vi "Edge Detection-2.vi"(8 "error in":errorcluster, 11 "Image":T1) -> (0 "error out":errorcluster, 1 "Particle Variables":i32[](array[ring]) items=["Center of Mass X", "Center of Mass Y", "First Pixel X", "First Pixel Y", "Bounding Rect Left", "Bounding Rect Top", "Bounding Rect Right", "Bounding Rect Bottom", "Max Feret Diameter Start X", "Max Feret Diameter Start Y", "Max Feret Diameter End X", "Max Feret Diameter End Y", "Max Horiz. Segment Length Left", "Max Horiz. Segment Length Right", "Max Horiz. Segment Length Row", "-", "Bounding Rect Width", "Bounding Rect Height", "Bounding Rect Diagonal", "Perimeter", "Convex Hull Perimeter", "Holes' Perimeter", "Max Feret Diameter", "Equivalent Ellipse Major Axis", "Equivalent Ellipse Minor Axis", "Equivalent Ellipse Minor Axis (Feret)", "Equivalent Rect Long Side", "Equivalent Rect Short Side", "Equivalent Rect Diagonal", "Equivalent Rect Short Side (Feret)", "Average Horiz. Segment Length", "Average Vert. Segment Length", "Hydraulic Radius", "Waddel Disk Diameter", "-", "Area", "Holes' Area", "Particle & Holes' Area", "Convex Hull Area", "Image Area", "-", "Number of Holes", "Number of Horiz. Segments", "Number of Vert. Segments", "-", "Orientation", "Max Feret Diameter Orientation", "-", "% Area/Image Area", "% Area/(Particle & Holes' Area)", "Ratio of Equivalent Ellipse Axes", "Ratio of Equivalent Rect Sides", "-", "Elongation Factor", "Compactness Factor", "Heywood Circularity Factor", "Type Factor", "-", "Sum X", "Sum Y", "Sum XX", "Sum XY", "Sum YY", "Sum XXX", "Sum XXY", "Sum XYY", "Sum YYY", "-", "Moment of Inertia XX", "Moment of Inertia XY", "Moment of Inertia YY", "Moment of Inertia XXX", "Moment of Inertia XXY", "Moment of Inertia XYY", "Moment of Inertia YYY", "Norm. Moment of Inertia XX", "Norm. Moment of Inertia XY", "Norm. Moment of Inertia YY", "Norm. Moment of Inertia XXX", "Norm. Moment of Inertia XXY", "Norm. Moment of Inertia XYY", "Norm. Moment of Inertia YYY", "Hu Moment 1", "Hu Moment 2", "Hu Moment 3", "Hu Moment 4", "Hu Moment 5", "Hu Moment 6", "Hu Moment 7"], 2 "Particle Measurements (Pixels)":dbl[][](array[numeric]) format="%.2f", 3 "Image Out":T1(plugin-control), 5 "Number of Particles":i32)   [LabVIEW 2014]
uses:
  <vilib>/vision/Image Controls.llb/IMAQ Image.ctl
  <vilib>/vision/Measure.llb/Edge Options.ctl
  <vilib>/vision/Measure.llb/Edge Polarity.ctl
  FileIO/TypeDef - File Actions.ctl
  <vilib>/vision/NI_Vision_Development_Module.lvlib
panel:
  in  "Display delay (s)":dbl min=0.0 max=5.0 step=0.5
  out "Task":string
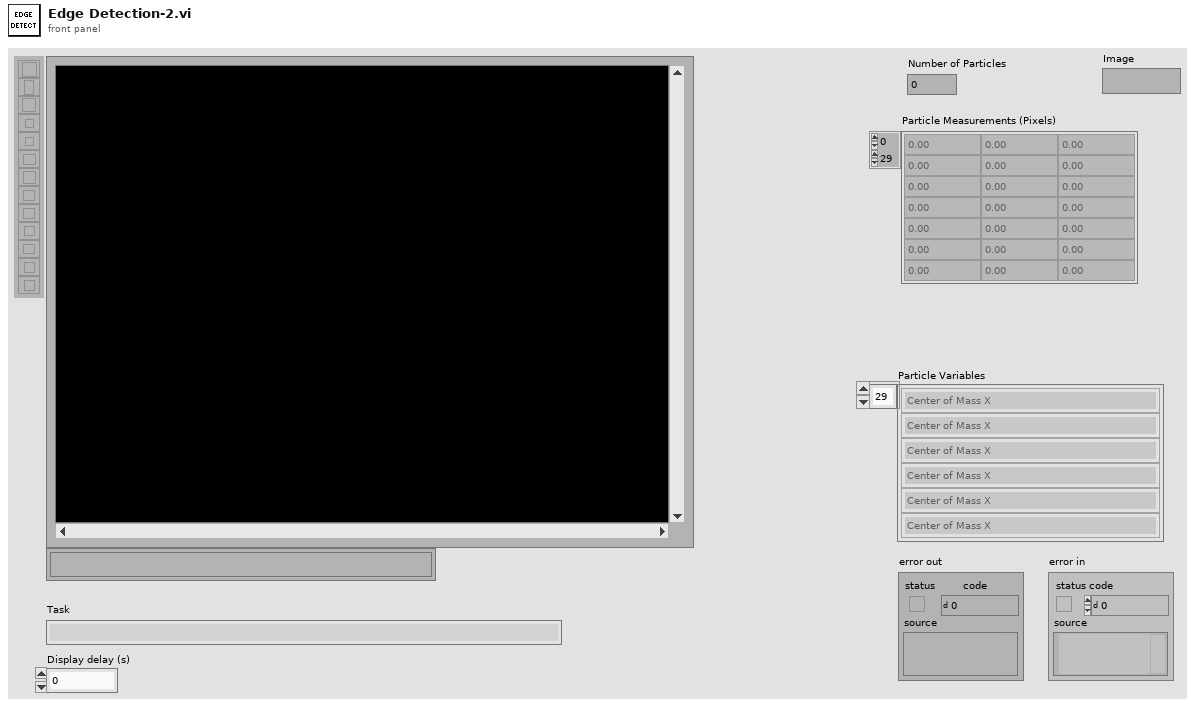
[diagram p1: front panel]
types:
  T1 = typedef "IMAQ Image.ctl" = refnum<image>
  T2 = enum32{"AutoM", "Close", "Dilate", "Erode", "Gradient", "Gradient out", "Gradient in", "Hit miss", "Open", "PClose", "POpen", "Thick", "Thin"}
  T3 = typedef "TypeDef - File Actions.ctl" = enum16{"Read", "Write", "Get Current"}
  T4 = cluster{"Measurement Parameter":i32, "Range Lower Value":dbl, "Range Upper Value":dbl, "Range":bool, "Measurement Type":bool}
  T5 = typedef "Image Type" = u32
  T6 = typedef "Edge Options.ctl" = cluster{"Edge Polarity":T7, "Kernel Size":u32, "Width":u32, "Minimum Edge Strength":sgl, "Interpolation Type":enum32{"Zero Order", "Bilinear", "Quadratic", "Cubic", "Bilinear Fixed"}, "Data Processing Method":enum32{"Average", "Median"}}
  T7 = typedef "Edge Polarity.ctl" = u32
  T8 = cluster{"Search  Direction":u32, "Edge Options":T6, "Show Search Area":bool, "Show Search Lines":bool, "Show Edges Found":bool, "Show Result":bool, "Search Area Color":u32, "Search Lines Color":u32, "Edge Locations Color":u32, "Result Color":u32, "Overlay Group Name":string}
  T9 = cluster{"Process":enum16{"Get First Edge", "Get First + Last Edge", "Get All Edges", "Get Best Edge"}, "Step Size":i32, "Max Pixel Radius":i32}
  T10 = cluster{"Global Rectangle":i32[], "Contours":cluster{"ID":enum32{"External", "Internal"}, "Type":u32, "Coordinates":i32[]}[]}
  T11 = enum32{"Differentiation", "Gradient", "Prewitt", "Roberts", "Sigma", "Sobel"}
  T12 = enum32{"Invalid", "Standard", "Closed", "Hidden", "Minimized", "Maximized"}
  T13 = typedef "TypeDef - System Configuration.ctl" = cluster{"Results FilePath":path, "Analysis Parameters":cluster{"Area":cluster{"Lower Value":dbl, "Upper Value":dbl}, "Circle Filter Radius":cluster{"Lower Value":sgl, "Upper Value":sgl}, "Edge Detection Threshold":u16}, "ROI Parameters":cluster{"ROI size (in Radius)":cluster{"Width":dbl, "Height":dbl}}}
  T14 = cluster{"Center (Pixels)":cluster{"X":sgl, "Y":sgl}, "Radius (Pixels)":dbl, "Center (Real-World)":cluster{"X":sgl, "Y":sgl}, "Radius (Real-World)":dbl, "Roundness (Real-World)":dbl, "Average Strength":dbl, "Average SNR (dB)":dbl}
  T15 = cluster{"Measurement Parameter":i32, "Range Lower Value":dbl, "Range Upper Value":dbl, "Range":bool, "Measurement Type":bool}[]
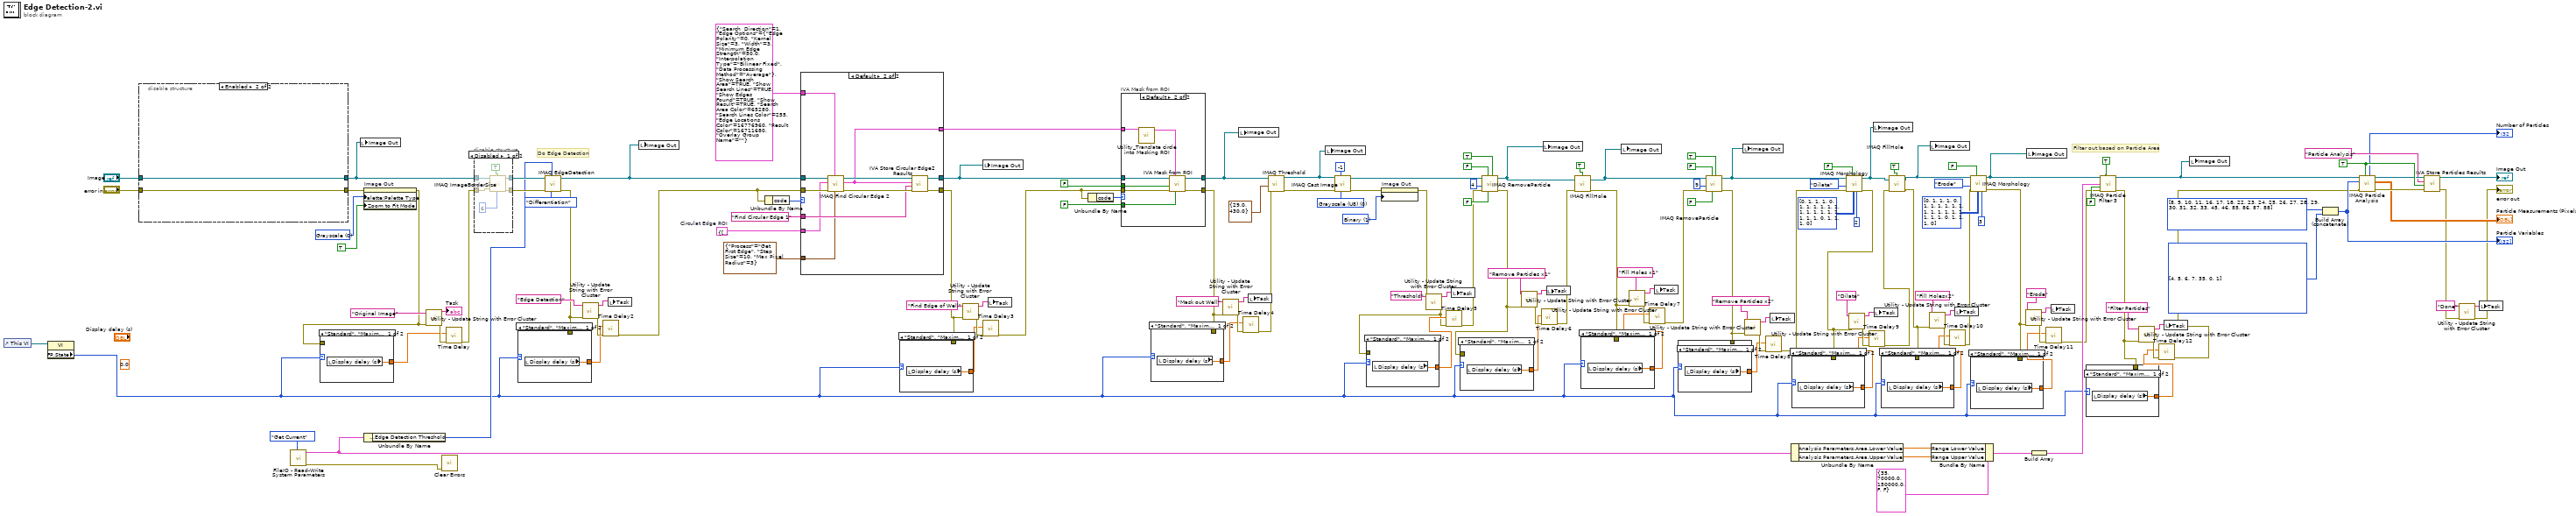
[diagram p0: block diagram]
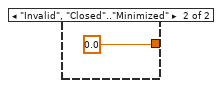
[diagram p2: hidden frame]
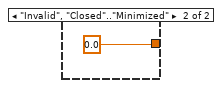
[diagram p3: hidden frame]
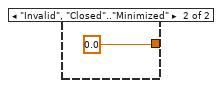
[diagram p4: hidden frame]
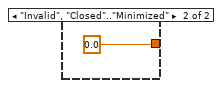
[diagram p5: hidden frame]
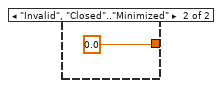
[diagram p6: hidden frame]
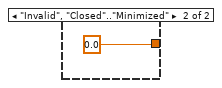
[diagram p7: hidden frame]
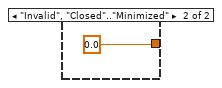
[diagram p8: hidden frame]
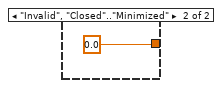
[diagram p9: hidden frame]
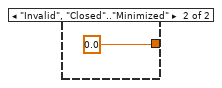
[diagram p10: hidden frame]
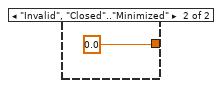
[diagram p11: hidden frame]
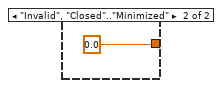
[diagram p12: hidden frame]
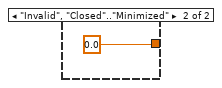
[diagram p13: hidden frame]
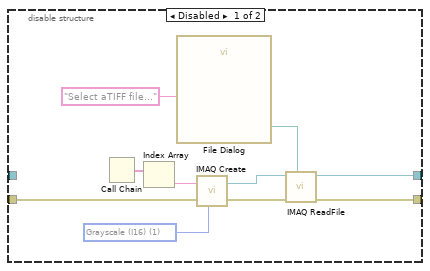
[diagram p16: hidden frame]
diagram:
  (unwired) 0.0 ("f")
  w108 = i32[] [4, 5, 6, 7, 35, 0, 1] items=["Center of Mass X", "Center of Mass Y", "First Pixel X", "First Pixel Y", "Bounding Rect Left", "Bounding Rect Top", "Bounding Rect Right", "Bounding Rect Bottom", "Max Feret Diameter Start X", "Max Feret Diameter Start Y", "Max Feret Diameter End X", "Max Feret Diameter End Y", "Max Horiz. Segment Length Left", "Max Horiz. Segment Length Right", "Max Horiz. Segment Length Row", "-", "Bounding Rect Width", "Bounding Rect Height", "Bounding Rect Diagonal", "Perimeter", "Convex Hull Perimeter", "Holes' Perimeter", "Max Feret Diameter", "Equivalent Ellipse Major Axis", "Equivalent Ellipse Minor Axis", "Equivalent Ellipse Minor Axis (Feret)", "Equivalent Rect Long Side", "Equivalent Rect Short Side", "Equivalent Rect Diagonal", "Equivalent Rect Short Side (Feret)", "Average Horiz. Segment Length", "Average Vert. Segment Length", "Hydraulic Radius", "Waddel Disk Diameter", "-", "Area", "Holes' Area", "Particle & Holes' Area", "Convex Hull Area", "Image Area", "-", "Number of Holes", "Number of Horiz. Segments", "Number of Vert. Segments", "-", "Orientation", "Max Feret Diameter Orientation", "-", "% Area/Image Area", "% Area/(Particle & Holes' Area)", "Ratio of Equivalent Ellipse Axes", "Ratio of Equivalent Rect Sides", "-", "Elongation Factor", "Compactness Factor", "Heywood Circularity Factor", "Type Factor", "-", "Sum X", "Sum Y", "Sum XX", "Sum XY", "Sum YY", "Sum XXX", "Sum XXY", "Sum XYY", "Sum YYY", "-", "Moment of Inertia XX", "Moment of Inertia XY", "Moment of Inertia YY", "Moment of Inertia XXX", "Moment of Inertia XXY", "Moment of Inertia XYY", "Moment of Inertia YYY", "Norm. Moment of Inertia XX", "Norm. Moment of Inertia XY", "Norm. Moment of Inertia YY", "Norm. Moment of Inertia XXX", "Norm. Moment of Inertia XXY", "Norm. Moment of Inertia XYY", "Norm. Moment of Inertia YYY", "Hu Moment 1", "Hu Moment 2", "Hu Moment 3", "Hu Moment 4", "Hu Moment 5", "Hu Moment 6", "Hu Moment 7"] ("Pixel Measurements")
  w111 = u32 0 items=["Grayscale", "Binary", "Gradient", "Rainbow", "Temperature", "User Defined"] ("Palette")
  w121 = u32 1 items=["Grayscale", "Binary", "Gradient", "Rainbow", "Temperature", "User Defined"] ("Palette")
  w109 = i32[] [8, 9, 10, 11, 16, 17, 18, 22, 23, 24, 25, 26, 27, 28, 29, 30, 31, 32, 33, 45, 46, 85, 86, 87, 88] items=["Center of Mass X", "Center of Mass Y", "First Pixel X", "First Pixel Y", "Bounding Rect Left", "Bounding Rect Top", "Bounding Rect Right", "Bounding Rect Bottom", "Max Feret Diameter Start X", "Max Feret Diameter Start Y", "Max Feret Diameter End X", "Max Feret Diameter End Y", "Max Horiz. Segment Length Left", "Max Horiz. Segment Length Right", "Max Horiz. Segment Length Row", "-", "Bounding Rect Width", "Bounding Rect Height", "Bounding Rect Diagonal", "Perimeter", "Convex Hull Perimeter", "Holes' Perimeter", "Max Feret Diameter", "Equivalent Ellipse Major Axis", "Equivalent Ellipse Minor Axis", "Equivalent Ellipse Minor Axis (Feret)", "Equivalent Rect Long Side", "Equivalent Rect Short Side", "Equivalent Rect Diagonal", "Equivalent Rect Short Side (Feret)", "Average Horiz. Segment Length", "Average Vert. Segment Length", "Hydraulic Radius", "Waddel Disk Diameter", "-", "Area", "Holes' Area", "Particle & Holes' Area", "Convex Hull Area", "Image Area", "-", "Number of Holes", "Number of Horiz. Segments", "Number of Vert. Segments", "-", "Orientation", "Max Feret Diameter Orientation", "-", "% Area/Image Area", "% Area/(Particle & Holes' Area)", "Ratio of Equivalent Ellipse Axes", "Ratio of Equivalent Rect Sides", "-", "Elongation Factor", "Compactness Factor", "Heywood Circularity Factor", "Type Factor", "-", "Sum X", "Sum Y", "Sum XX", "Sum XY", "Sum YY", "Sum XXX", "Sum XXY", "Sum XYY", "Sum YYY", "-", "Moment of Inertia XX", "Moment of Inertia XY", "Moment of Inertia YY", "Moment of Inertia XXX", "Moment of Inertia XXY", "Moment of Inertia XYY", "Moment of Inertia YYY", "Norm. Moment of Inertia XX", "Norm. Moment of Inertia XY", "Norm. Moment of Inertia YY", "Norm. Moment of Inertia XXX", "Norm. Moment of Inertia XXY", "Norm. Moment of Inertia XYY", "Norm. Moment of Inertia YYY", "Hu Moment 1", "Hu Moment 2", "Hu Moment 3", "Hu Moment 4", "Hu Moment 5", "Hu Moment 6", "Hu Moment 7"] ("Pixel Measurements")
  w125 = TRUE ("Connectivity 4/8 (8)")
  w141 = T5 0 items=["Grayscale (U8)", "Grayscale (I16)", "Grayscale (SGL)", "Complex (CSG)", "RGB (U32)", "HSL (U32)", "RGB (U64)", "Grayscale (U16)"] ("Image Type")
  w148 = T10 {"Global Rectangle"=[18, -169, 2540, 2352], "Contours"=[{"ID"=enum."External", "Type"=7, "Coordinates"=[1278, 1091, 691, 1260, 0, 359834]}]}  # Circulat Edge ROI
  # "Do Edge Detection"
  # "Filter out based on Particle Area"
  n1 = control-ref of="This VI"() -> (w80:refnum<vi>)
  n2 = property class="VI"(reference=w80) -> ("FP.State"=w3:T12)  [unwired: 1 in, 2 out]
  n3 = disable-structure shown="Enabled" {
    disable-tunnel: [w163 w165] -> w104
    disable-tunnel: "error in" -> [w161 w165]
    disable-tunnel: [w155 w164] -> w120
    disable-tunnel: "Image" -> [_ w164]
    frame Disabled {
      w156 = T5 1 items=["Grayscale (U8)", "Grayscale (I16)", "Grayscale (SGL)", "Complex (CSG)", "RGB (U32)", "HSL (U32)", "RGB (U64)", "Grayscale (U16)"] ("Image Type")
      n4 = Call Chain() -> (call chain=w160:string[])
      n5 = Index Array(array=w160) -> (element=w159:string)  [unwired: 1 in]
      n6 = call "File Dialog"("prompt"="Select aTIFF file...") -> ("selected path"=w157:path)  [unwired: 6 in, 8 out]
      n7 = call "IMAQ Create"("Image Name"=w159, "Image Type"=w156, "error in (no error)"=w161) -> ("New Image"=w162:T1, "error out"=w154:errorcluster)  [unwired: 1 in, 1 out]
      n8 = call "IMAQ ReadFile"("File Path"=w157, "error in (no error)"=w154, "Image"=w162) -> ("error out"=w163:errorcluster, "Image Out"=w155:T1)  [unwired: 2 in, 5 out]
    }
    frame Enabled {
    }
  }
  n9 = call "FileIO - Read-Write System Parameters.vi"("Action"=TypeDef_-_File_Actions."Get Current") -> ("error out"=w96:errorcluster, "System Parameters out"=w18:T13)  [unwired: 9 in]
  n10 = local write "Image Out"(w120) -> ()
  n11 = property on="Image Out" class="ImageControl"(error in=w104, "Palette:Palette Type"=w111, "Zoom to Fit Mode"=TRUE) -> (error out=w27:errorcluster)  [unwired: 1 in, 1 out]
  n12 = case shown="\"Standard\", \"Maximized\"" w3 {
    tunnel: [w166 0.0 ("f")] -> w26
    tunnel: w27 -> [_ _]
    frame "Standard", "Maximized" {
      n13 = local read "Display delay (s)"() -> (w166:dbl)
    }
    frame "Invalid", "Closed".."Minimized" {
    }
  }
  n14 = Unbundle By Name(w18) -> ("Analysis Parameters.Edge Detection Threshold"=w16:u16)
  n15 = call "Utility - Update String with Error Cluster.vi"("error in (no error)"=w27, "String In"="Original Image" ("Task")) -> ("error out"=w76:errorcluster, "String Out"=→"Task":string)  [unwired: 8 in]
  n16 = call <vilib>:"Clear Errors.vi"("error in (no error)"=w96) -> ()  [unwired: 5 in, 2 out]
  n17 = call "Time Delay"("error in (no error)"=w76, "Delay Time (s)"=w26) -> ("error out"=w79:errorcluster)  [unwired: 9 in]
  n18 = disable-structure shown="Disabled" {
    disable-tunnel: [w173 w174] -> w152
    disable-tunnel: [w170 w175] -> w150
    disable-tunnel: w120 -> [w169 w175]
    disable-tunnel: w79 -> [w168 w174]
    frame Disabled {
      n19 = call "IMAQ ImageBorderSize"("Get/Set Status? (Set)"=TRUE, "Image"=w169, "Image border size in"=6 ("Border Size"), "error in (no error)"=w168) -> ("Image Out"=w170:T1, "error out"=w173:errorcluster)  [unwired: 1 out]
    }
    frame Enabled {
    }
  }
  n20 = call "IMAQ EdgeDetection"("Method"=T11."Differentiation", "Threshold Value"=w16, "error in (no error)"=w152, "Image Src"=w150) -> ("error out"=w25:errorcluster, "Image Dst Out"=w119:T1)  [unwired: 2 in, 4 out]
  n21 = case shown="\"Standard\", \"Maximized\"" w3 {
    tunnel: [w176 0.0 ("f")] -> w17
    tunnel: w25 -> [_ _]
    frame "Standard", "Maximized" {
      n22 = local read "Display delay (s)"() -> (w176:dbl)
    }
    frame "Invalid", "Closed".."Minimized" {
    }
  }
  n23 = call "Utility - Update String with Error Cluster.vi"("error in (no error)"=w25, "String In"="Edge Detection") -> ("error out"=w75:errorcluster, "String Out"=w73:string)  [unwired: 8 in]
  n24 = call "Time Delay2"("error in (no error)"=w75, "Delay Time (s)"=w17) -> ("error out"=w74:errorcluster)  [unwired: 9 in]
  n25 = local write "Task"(w73) -> ()
  n26 = local write "Image Out"(w119) -> ()
  n27 = Unbundle By Name(w74) -> ("code"=w147:i32)
  n28 = case shown="Default" w147 {
    tunnel: T8 {"Search  Direction"=1, "Edge Options"={"Edge Polarity"=0, "Kernel Size"=3, "Width"=3, "Minimum Edge Strength"=50.0, "Interpolation Type"=enum."Bilinear Fixed", "Data Processing Method"=enum."Average"}, "Show Search Area"=TRUE, "Show Search Lines"=TRUE, "Show Edges Found"=TRUE, "Show Result"=TRUE, "Search Area Color"=65280, "Search Lines Color"=255, "Edge Locations Color"=16776960, "Result Color"=16711680, "Overlay Group Name"=""} ("Options") -> [_ w179]
    tunnel: w119 -> [w178 w189]
    tunnel: w74 -> [_ w188]
    tunnel: [_ w186] -> w23
    tunnel: [w178 w184] -> w118
    tunnel: "Find Circular Edge 1" ("Step Name") -> [_ w183]
    tunnel: w148 -> [_ w182]
    tunnel: T9 {"Process"=enum."Get First Edge", "Step Size"=10, "Max Pixel Radius"=3} ("Circle Fit Options") -> [_ w181]
    tunnel: [_ w180] -> w90
    frame -1074396199, -1074396198 {
      # "Discard Coordinate System Error"
    }
    frame Default {
      n29 = call "IMAQ Find Circular Edge 2"("Circle Fit Options"=w181, "Options"=w179, "error in (no error)"=w188, "ROI Descriptor"=w182, "Image"=w189) -> ("error out"=w187:errorcluster, "Fitted Circle"=w180:T14, "Image Out"=w185:T1)  [unwired: 1 in, 3 out]
      n30 = call <vilib>:"IVA Store Circular Edge2 Results.vi"("error in (no error)"=w187, "Step Name"=w183, "Fitted Circle"=w180, "Image in"=w185) -> ("error out"=w186:errorcluster, "Image dup"=w184:T1)  [unwired: 2 in, 4 out]
    }
  }
  n31 = case shown="\"Standard\", \"Maximized\"" w3 {
    tunnel: [w190 0.0 ("f")] -> w24
    tunnel: w23 -> [_ _]
    frame "Standard", "Maximized" {
      n32 = local read "Display delay (s)"() -> (w190:dbl)
    }
    frame "Invalid", "Closed".."Minimized" {
    }
  }
  n33 = call "Utility - Update String with Error Cluster.vi"("error in (no error)"=w23, "String In"="Find Edge of Well") -> ("error out"=w70:errorcluster, "String Out"=w71:string)  [unwired: 8 in]
  n34 = local write "Image Out"(w118) -> ()
  n35 = call "Time Delay3"("error in (no error)"=w70, "Delay Time (s)"=w24) -> ("error out"=w69:errorcluster)  [unwired: 9 in]
  n36 = local write "Task"(w71) -> ()
  n37 = Unbundle By Name(w69) -> ("code"=w91:i32)
  n38 = case "IVA Mask from ROI" shown="Default" w91 {
    tunnel: w90 -> [_ w194]
    tunnel: FALSE ("Shrink") -> [_ w200]
    tunnel: w118 -> [w192 w199]
    tunnel: w69 -> [_ w198]
    tunnel: [_ w197] -> w22
    tunnel: [w192 w196] -> w117
    tunnel: FALSE ("Out / In") -> [_ w195]
    frame -1074396199, -1074396198 {
      # "Discard\nCoordinate\nSystem\nError"
    }
    frame Default {
      n39 = call "Utility_Translate circle into Masking ROI.vi"("Fitted Circle"=w194) -> ("ROI Descriptor"=w193:T10)  [unwired: 10 in]
      n40 = call <vilib>:"IVA Mask from ROI.vi"("Shrink"=w200, "ROI Descriptor"=w193, "error in (no error)"=w198, "Out / In"=w195, "Image Src"=w199) -> ("error out"=w197:errorcluster, "Image Out"=w196:T1)  [unwired: 5 out]
    }
  }
  n41 = case shown="\"Standard\", \"Maximized\"" w3 {
    tunnel: [w201 0.0 ("f")] -> w21
    tunnel: w22 -> [_ _]
    frame "Standard", "Maximized" {
      n42 = local read "Display delay (s)"() -> (w201:dbl)
    }
    frame "Invalid", "Closed".."Minimized" {
    }
  }
  n43 = call "Utility - Update String with Error Cluster.vi"("error in (no error)"=w22, "String In"="Mask out Well") -> ("error out"=w66:errorcluster, "String Out"=w65:string)  [unwired: 8 in]
  n44 = local write "Image Out"(w117) -> ()
  n45 = call "Time Delay4"("error in (no error)"=w66, "Delay Time (s)"=w21) -> ("error out"=w64:errorcluster)  [unwired: 9 in]
  n46 = local write "Task"(w65) -> ()
  n47 = call "IMAQ Threshold"("error in (no error)"=w64, "Range"=cluster{"Lower value":sgl, "Upper value":sgl} {"Lower value"=29.0, "Upper value"=430.0}, "Image Src"=w117) -> ("error out"=w143:errorcluster, "Image Dst Out"=w116:T1)  [unwired: 3 in, 4 out]
  n48 = local write "Image Out"(w116) -> ()
  n49 = call "IMAQ Cast Image"("Image Type"=w141, "# Shifts"=-1, "error in (no error)"=w143, "Image Src"=w116) -> ("error out"=w110:errorcluster, "Image Dst Out"=w136:T1)  [unwired: 2 in, 4 out]
  n50 = property on="Image Out" class="ImageControl"(error in=w110, "Palette:Palette Type"=w121) -> (error out=w61:errorcluster)  [unwired: 1 in, 1 out]
  n51 = call "Utility - Update String with Error Cluster.vi"("error in (no error)"=w61, "String In"="Threshold") -> ("error out"=w19:errorcluster, "String Out"=w63:string)  [unwired: 8 in]
  n52 = case shown="\"Standard\", \"Maximized\"" w3 {
    tunnel: [w203 0.0 ("f")] -> w20
    tunnel: w19 -> [_ _]
    frame "Standard", "Maximized" {
      n53 = local read "Display delay (s)"() -> (w203:dbl)
    }
    frame "Invalid", "Closed".."Minimized" {
    }
  }
  n54 = call "Time Delay5"("error in (no error)"=w19, "Delay Time (s)"=w20) -> ("error out"=w60:errorcluster)  [unwired: 9 in]
  n55 = local write "Task"(w63) -> ()
  n56 = call "IMAQ RemoveParticle"("Connectivity 4/8 (8)"=TRUE, "Low Pass/High Pass (Low)"=FALSE, "Square/Hexa (Square)"=FALSE, "error in (no error)"=w60, "Number of Erosion"=4, "Image Src"=w136) -> ("error out"=w15:errorcluster, "Image Dst Out"=w115:T1)  [unwired: 1 in, 3 out]
  n57 = case shown="\"Standard\", \"Maximized\"" w3 {
    tunnel: [w205 0.0 ("f")] -> w14
    tunnel: w15 -> [_ _]
    frame "Standard", "Maximized" {
      n58 = local read "Display delay (s)"() -> (w205:dbl)
    }
    frame "Invalid", "Closed".."Minimized" {
    }
  }
  n59 = call "Utility - Update String with Error Cluster.vi"("error in (no error)"=w15, "String In"="Remove Particles x1") -> ("error out"=w58:errorcluster, "String Out"=w57:string)  [unwired: 8 in]
  n60 = call "Time Delay6"("error in (no error)"=w58, "Delay Time (s)"=w14) -> ("error out"=w56:errorcluster)  [unwired: 9 in]
  n61 = local write "Image Out"(w115) -> ()
  n62 = local write "Task"(w57) -> ()
  n63 = call "IMAQ FillHole"("error in (no error)"=w56, "Image Src"=w115, "Connectivity 4/8 (8)"=TRUE) -> ("error out"=w12:errorcluster, "Image Dst Out"=w114:T1)  [unwired: 1 in, 2 out]
  n64 = case shown="\"Standard\", \"Maximized\"" w3 {
    tunnel: [w207 0.0 ("f")] -> w13
    tunnel: w12 -> [_ _]
    frame "Standard", "Maximized" {
      n65 = local read "Display delay (s)"() -> (w207:dbl)
    }
    frame "Invalid", "Closed".."Minimized" {
    }
  }
  n66 = local write "Image Out"(w114) -> ()
  n67 = call "Utility - Update String with Error Cluster.vi"("error in (no error)"=w12, "String In"="Fill Holes x1") -> ("error out"=w54:errorcluster, "String Out"=w55:string)  [unwired: 8 in]
  n68 = call "Time Delay7"("error in (no error)"=w54, "Delay Time (s)"=w13) -> ("error out"=w52:errorcluster)  [unwired: 9 in]
  n69 = local write "Task"(w55) -> ()
  n70 = call "IMAQ RemoveParticle"("Connectivity 4/8 (8)"=TRUE, "Low Pass/High Pass (Low)"=FALSE, "Square/Hexa (Square)"=FALSE, "error in (no error)"=w52, "Number of Erosion"=9, "Image Src"=w114) -> ("error out"=w11:errorcluster, "Image Dst Out"=w113:T1)  [unwired: 1 in, 3 out]
  n71 = case shown="\"Standard\", \"Maximized\"" w3 {
    tunnel: [w209 0.0 ("f")] -> w10
    tunnel: w11 -> [_ _]
    frame "Standard", "Maximized" {
      n72 = local read "Display delay (s)"() -> (w209:dbl)
    }
    frame "Invalid", "Closed".."Minimized" {
    }
  }
  n73 = local write "Image Out"(w113) -> ()
  n74 = call "Utility - Update String with Error Cluster.vi"("error in (no error)"=w11, "String In"="Remove Particles x2") -> ("error out"=w50:errorcluster, "String Out"=w49:string)  [unwired: 8 in]
  n75 = call "Time Delay8"("error in (no error)"=w50, "Delay Time (s)"=w10) -> ("error out"=w48:errorcluster)  [unwired: 9 in]
  n76 = local write "Task"(w49) -> ()
  n77 = Unbundle By Name(w18) -> ("Analysis Parameters.Area.Lower Value"=w98:dbl, "Analysis Parameters.Area.Upper Value"=w97:dbl)
  n78 = call "IMAQ Morphology"("Number of iterations (1)"=2, "Structuring Element"=i32[][] [[0, 1, 1, 1, 0], [1, 1, 1, 1, 1], [1, 1, 1, 1, 1], [1, 1, 1, 1, 1], [0, 1, 1, 1, 0]], "Square/Hexa (Square)"=FALSE, "error in (no error)"=w48, "Operation"=T2."Dilate", "Image Src"=w113) -> ("error out"=w8:errorcluster, "Image Dst Out"=w83:T1)  [unwired: 1 in, 3 out]
  n79 = case shown="\"Standard\", \"Maximized\"" w3 {
    tunnel: [w211 0.0 ("f")] -> w9
    tunnel: w8 -> [_ _]
    frame "Standard", "Maximized" {
      n80 = local read "Display delay (s)"() -> (w211:dbl)
    }
    frame "Invalid", "Closed".."Minimized" {
    }
  }
  n81 = call "Utility - Update String with Error Cluster.vi"("error in (no error)"=w8, "String In"="Dilate") -> ("error out"=w46:errorcluster, "String Out"=w47:string)  [unwired: 8 in]
  n82 = call "Time Delay9"("error in (no error)"=w46, "Delay Time (s)"=w9) -> ("error out"=w44:errorcluster)  [unwired: 9 in]
  n83 = local write "Image Out"(w83) -> ()
  n84 = local write "Task"(w47) -> ()
  n85 = call "IMAQ FillHole"("error in (no error)"=w44, "Image Src"=w83, "Connectivity 4/8 (8)"=TRUE) -> ("error out"=w6:errorcluster, "Image Dst Out"=w82:T1)  [unwired: 1 in, 2 out]
  n86 = case shown="\"Standard\", \"Maximized\"" w3 {
    tunnel: [w213 0.0 ("f")] -> w7
    tunnel: w6 -> [_ _]
    frame "Standard", "Maximized" {
      n87 = local read "Display delay (s)"() -> (w213:dbl)
    }
    frame "Invalid", "Closed".."Minimized" {
    }
  }
  n88 = call "Utility - Update String with Error Cluster.vi"("error in (no error)"=w6, "String In"="Fill Holesx2") -> ("error out"=w42:errorcluster, "String Out"=w41:string)  [unwired: 8 in]
  n89 = local write "Image Out"(w82) -> ()
  n90 = Bundle By Name(cluster=T4 {"Measurement Parameter"=35, "Range Lower Value"=70000.0, "Range Upper Value"=150000.0, "Range"=FALSE, "Measurement Type"=FALSE} ("Selection Value"), "Range Lower Value"=w98, "Range Upper Value"=w97) -> (w89:T4)
  n91 = call "Time Delay10"("error in (no error)"=w42, "Delay Time (s)"=w7) -> ("error out"=w40:errorcluster)  [unwired: 9 in]
  n92 = local write "Task"(w41) -> ()
  n93 = call "IMAQ Morphology"("Number of iterations (1)"=3, "Structuring Element"=i32[][] [[0, 1, 1, 1, 0], [1, 1, 1, 1, 1], [1, 1, 1, 1, 1], [1, 1, 1, 1, 1], [0, 1, 1, 1, 0]], "Square/Hexa (Square)"=FALSE, "error in (no error)"=w40, "Operation"=T2."Erode", "Image Src"=w82) -> ("error out"=w4:errorcluster, "Image Dst Out"=w84:T1)  [unwired: 1 in, 3 out]
  n94 = case shown="\"Standard\", \"Maximized\"" w3 {
    tunnel: [w215 0.0 ("f")] -> w5
    tunnel: w4 -> [_ _]
    frame "Standard", "Maximized" {
      n95 = local read "Display delay (s)"() -> (w215:dbl)
    }
    frame "Invalid", "Closed".."Minimized" {
    }
  }
  n96 = call "Utility - Update String with Error Cluster.vi"("error in (no error)"=w4, "String In"="Erode") -> ("error out"=w38:errorcluster, "String Out"=w39:string)  [unwired: 8 in]
  n97 = local write "Image Out"(w84) -> ()
  n98 = Build Array(w89) -> (w100:T15)
  n99 = call "Time Delay11"("error in (no error)"=w38, "Delay Time (s)"=w5) -> ("error out"=w34:errorcluster)  [unwired: 9 in]
  n100 = local write "Task"(w39) -> ()
  n101 = call "IMAQ Particle Filter 3"("Image Src"=w84, "Connectivity 4/8 (8)"=TRUE, "Selection Values"=w100, "Keep/Remove Particles (F)"=FALSE ("Keep/Remove Particles"), "error in (no error)"=w34) -> ("Image Dst Out"=w95:T1, "error out"=w2:errorcluster)  [unwired: 4 in, 5 out]
  n102 = case shown="\"Standard\", \"Maximized\"" w3 {
    tunnel: [w217 0.0 ("f")] -> w1
    tunnel: w2 -> [_ _]
    frame "Standard", "Maximized" {
      n103 = local read "Display delay (s)"() -> (w217:dbl)
    }
    frame "Invalid", "Closed".."Minimized" {
    }
  }
  n104 = call "Utility - Update String with Error Cluster.vi"("error in (no error)"=w2, "String In"="Filter Particles") -> ("error out"=w36:errorcluster, "String Out"=w35:string)  [unwired: 8 in]
  n105 = call "Time Delay12"("error in (no error)"=w36, "Delay Time (s)"=w1) -> ("error out"=w33:errorcluster)  [unwired: 9 in]
  n106 = local write "Task"(w35) -> ()
  n107 = local write "Image Out"(w95) -> ()
  n108 = Build Array (concatenate)(w109, w108) -> (w107:i32[])
  "Particle Variables" <- w107
  n109 = call "IMAQ Particle Analysis"("Connectivity 4/8 (8)"=w125, "error in (no error)"=w33, "Pixel Measurements"=w107, "Image"=w95) -> ("error out"=w122:errorcluster, "Particle Measurements (Pixels)"=→"Particle Measurements (Pixels)":dbl[][], "Image Out (duplicate)"=w124:T1, "Number of Particles"=→"Number of Particles":i32)  [unwired: 1 in, 3 out]
  n110 = call <vilib>:"IVA Store Particles Results.vi"("error in (no error)"=w122, "Connectivity 4/8 (8)"=w125, "Step Name"="Particle Analysis", "Image in"=w124) -> ("error out"=w31:errorcluster, "Image dup"=→"Image Out":T1)  [unwired: 6 out]
  n111 = call "Utility - Update String with Error Cluster.vi"("error in (no error)"=w31, "String In"="Done") -> ("error out"=→"error out":errorcluster, "String Out"=w30:string)  [unwired: 8 in]
  n112 = local write "Task"(w30) -> ()
